vi "new_from_dialect_and_contents.vi"(8 "error in (no error)":errorcluster, 9 "contents":string, 10 "dialect":string, 11 "OpaqueDialectType in":refnum<class "OpaqueDialectType.lvclass">) -> (0 "error out":errorcluster, 3 "OpaqueDialectType out":refnum<class "OpaqueDialectType.lvclass">)   [LabVIEW 2020, in "mlir.lvlib" / "OpaqueDialectType.lvclass"]
uses:
  OpaqueDialectType.lvclass
  OpaqueDialectType.lvclass/OpaqueDialectType.ctl
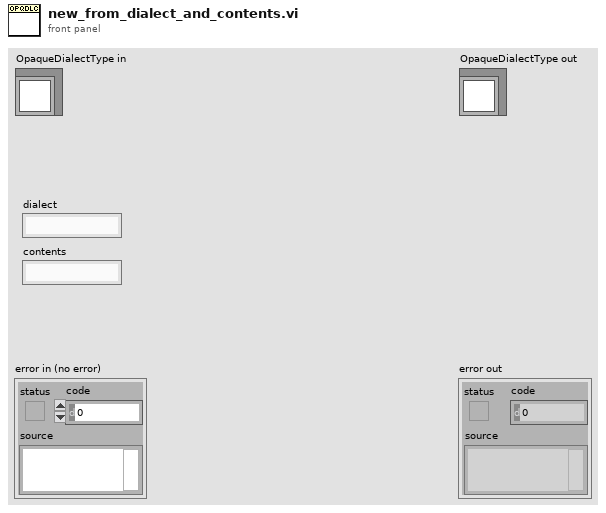
[diagram p1: front panel]
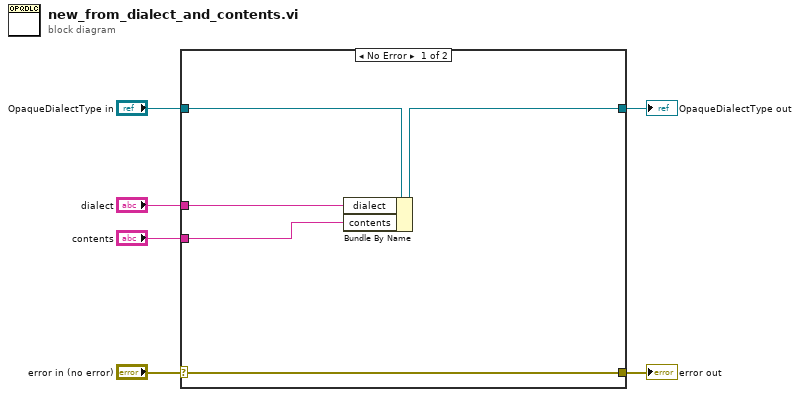
[diagram p0: block diagram]
diagram:
  n1 = case shown="No Error" "error in (no error)" {
    selector: "error in (no error)" -> [w10 w13]
    tunnel: [w10 w13] -> w5
    tunnel: [w9 w12] -> w3
    tunnel: "OpaqueDialectType in" -> [w11 w12]
    tunnel: "contents" -> [w8 _]
    tunnel: "dialect" -> [w7 _]
    frame No Error {
      n2 = Bundle By Name(cluster=w11, "dialect"=w7, "contents"=w8) -> (w9:refnum<class "OpaqueDialectType.lvclass">)
    }
    frame Error {
    }
  }
  "error out" <- w5
  "OpaqueDialectType out" <- w3
